vi "eliminatePositionRobot.vi"(10 "position(x,y)":dbl[](array[numeric]), 11 "5Positions":dbl[][](array[numeric])) -> (2 "deleted portion":dbl[](array[numeric]), 3 "sorted 2D array":dbl[][](array[numeric]))   [LabVIEW 2020, in "Ally.lvclass"]
uses:
  Ally.lvclass
  94447ec6-2117-4c56-b770-c52259c670bc.vi
  <vilib>/Array/Sort 2D Array - Pop Stack.vi
  <vilib>/Array/Sort 2D Array - Push Stack.vi
  94447ec6-2117-4c56-b770-c52259c670bc.vi/269d4b3b-47f5-49e3-8884-44851e4dd9d5.vi
  94447ec6-2117-4c56-b770-c52259c670bc.vi/6d99389c-673d-4efb-bf33-19b32bcf4cf8.vi
  Ally.lvclass/Ally.ctl
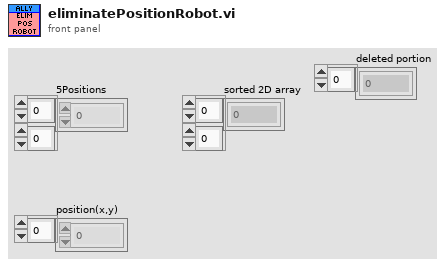
[diagram p1: front panel]
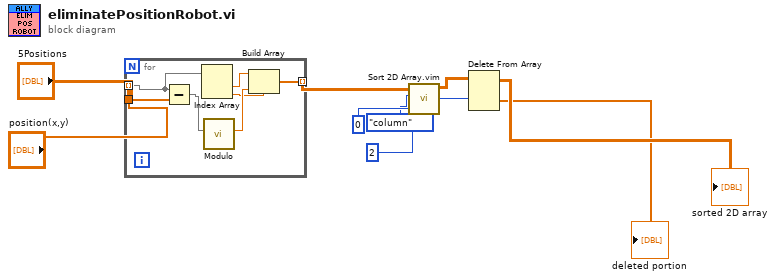
[diagram p0: block diagram]
diagram:
  n1 = for {
    tunnel: "5Positions" -> [w10] mode=indexing
    tunnel: "position(x,y)" -> [w16]
    tunnel: [w11] -> w2 mode=indexing
    n2 = Subtract(x=w10, y=w16) -> (x-y=w13:dbl[])
    n3 = Index Array(array=w10) -> (element #1=w14:dbl, element #2=w12:dbl)  [unwired: 2 in]
    n4 = call "Modulo.vi"("2D vector"=w13) -> ("Modulo"=w15:dbl)  [unwired: 10 in]
    n5 = Build Array(w14, w12, w15) -> (w11:dbl[])
  }
  n6 = call "Sort 2D Array.vim"("index"=2, "dimension to index (column)"=enum16{"column", "row"}."column", "2D array"=w2) -> ("sorted 2D array"=w5:dbl[][])  [unwired: 7 in, 1 out]
  n7 = Delete From Array(array=w5, index (row)=0) -> (deleted portion=→"deleted portion":dbl[], array with subset deleted=→"sorted 2D array":dbl[][])  [unwired: 2 in]
